vi "HEWH Select Master Flow Meter.vi"(8 "error in (no error)":errorcluster, 10 "Laurel Hot IP Address":string, 11 "Laurel Cold IP Address":string) -> (0 "error out":errorcluster, 2 "Flow Selector":T1, 3 "Master Flow Meter Address":string)   [LabVIEW 2020]
uses:
  Type Definitions/Flow Meter Selector.ctl
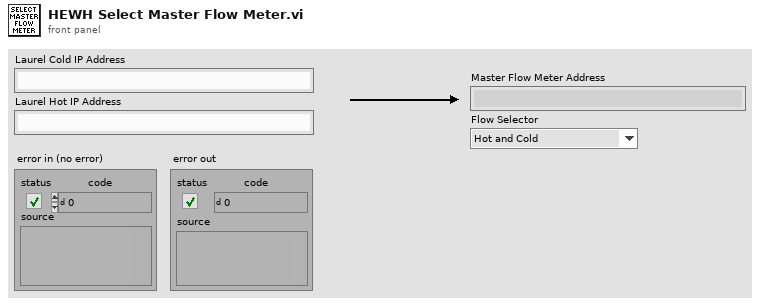
[diagram p1: front panel]
types:
  T1 = typedef "Flow Meter Selector.ctl" = enum16{"Hot and Cold", "Hot", "Cold", "None"}
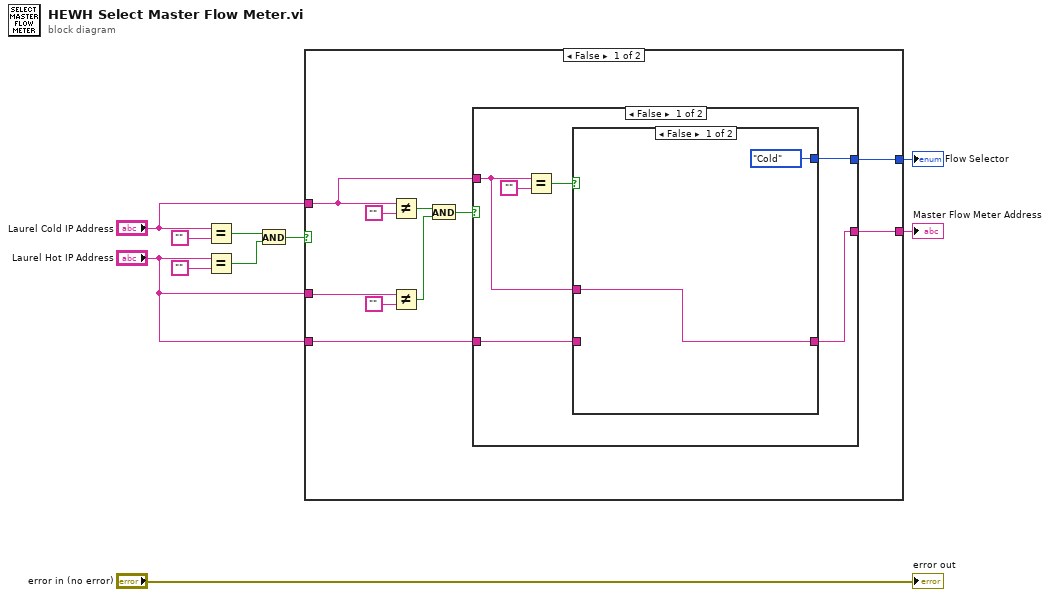
[diagram p0: block diagram]
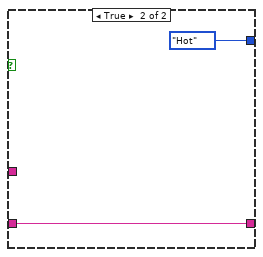
[diagram p2: hidden frame]
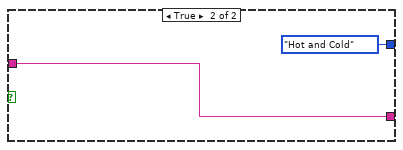
[diagram p3: hidden frame]
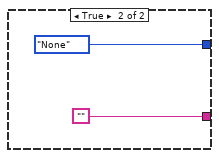
[diagram p4: hidden frame]
diagram:
  n1 = Equal?(x="Laurel Cold IP Address", y="") -> (x = y?=w8:bool)
  n2 = Equal?(x="Laurel Hot IP Address", y="") -> (x = y?=w7:bool)
  n3 = And(x=w8, y=w7) -> (x .and. y?=w6:bool)
  n4 = case shown="False" w6 {
    tunnel: [w20 ""] -> w4
    tunnel: "Laurel Cold IP Address" -> [w13 _]
    tunnel: "Laurel Hot IP Address" -> [w17 _]
    tunnel: "Laurel Hot IP Address" -> [w12 _]
    tunnel: [w11 Flow_Meter_Selector."None" ("Enum")] -> w1
    frame False {
      n5 = Not Equal?(x=w13, y="") -> (x != y?=w16:bool)
      n6 = Not Equal?(x=w17, y="") -> (x != y?=w15:bool)
      n7 = And(x=w16, y=w15) -> (x .and. y?=w14:bool)
      n8 = case shown="False" w14 {
        tunnel: [w23 w32] -> w20
        tunnel: w13 -> [w22 w32]
        tunnel: w12 -> [w24 _]
        tunnel: [w21 Flow_Meter_Selector."Hot and Cold" ("Enum")] -> w11
        frame False {
          n9 = Equal?(x=w22, y="") -> (x = y?=w25:bool)
          n10 = case shown="False" w25 {
            tunnel: w24 -> [_ w30]
            tunnel: [w28 w30] -> w23
            tunnel: w22 -> [w28 _]
            tunnel: [Flow_Meter_Selector."Cold" ("Enum") Flow_Meter_Selector."Hot" ("Enum")] -> w21
            frame False {
            }
            frame True {
            }
          }
        }
        frame True {
        }
      }
    }
    frame True {
    }
  }
  "Master Flow Meter Address" <- w4
  "Flow Selector" <- w1
  "error out" <- "error in (no error)"
